vi "Target Detection.vi"(0 "Camera Image":T1) -> (1 "Hot Vision Target":bool, 2 "Cold Vision Target":bool)   [LabVIEW 2013]
uses:
  Support/TargetType.ctl
  <vilib>/vision/Image Controls.llb/IMAQ Image.ctl
panel:
  out "loop time ms":u32
  in  "Instructions:":string="Images:\nUse the tab immediately below to choose the image source. Update the camera settings or the image directory so that you have images or video to test with.\n\nCalibration:\nYou can update Color Component ranges directly, or by clicking and drawing a line on the colored strip in the Image control. The Std Dev multipliers and where the strip is drawn determine the calibration values.\n\nUse Debugging tab to view the result of the color range threshold .\n\nArea Size LImit is used to ignore objects too small or far away to care about.\n\nThe Details tab contains score details for each target and subObject.\n\nCamera Type is used to select lens angles for distance calculation.\n\nVertical strips with no adjacent horizontal strip are identified as \"not hot\" and marked in blue.\nThe numeric scores indicate represent aspect ratio and rectangularity.\n\nWhen both strips are near enough, the pair is identified as \"hot\" and marked in green. Scores\nindicate the left, right, ratio of widths, and vertical positioning.\n\nAny score that falls below cutoff is drawn in red and bounding box is drawn in red."
  in  "Area Size Limit %":dbl=0.06 format="%#_13g"
  in  "Camera Type":enum16{"206", "1011", "1013"}(ring)=enum."1013"
  in  "Score Cutoff":dbl(slide)=54.248366013071895 scale=0.0..100.0
  in  "Color Components":T2={"Hue"={112.0, 144.0}, "Sat"={223.0, 255.0}, "Val"={237.0, 255.0}} {"Val" scale=0.0..255.0; "Sat" scale=0.0..255.0; "Hue" scale=0.0..255.0 scale format="%#_3g"}
  in  "Tabbed Info":enum32{"Debugging", "Details"}(tab)=enum."Details"
  out "Mask":T1(plugin-control)
  out "Target Info":T4(array[cluster])=[{"Scores"={"Total"=264.8428070737725, "Left"=82.00744831503384, "Right"=0.0, "Ratio"=95.56961423095669, "Vertical"=87.265744527782, "index"=0, "State"=enum."Hot"}, "Verticals"={"Horizontal?"=FALSE, "Aspect Score"=83.06845793962944, "Rect Score"=72.28571428571429, {"Left"=200.0, "Top"=96.0, "Right"=207.0, "Bottom"=146.0}, "Equiv H"=5.125465815260874, "Equiv V"=49.36136716524427}, "Horizontals"={"Horizontal?"=TRUE, "Aspect Score"=88.35576607935369, "Rect Score"=66.38655462184875, {"Left"=161.0, "Top"=90.0, "Right"=195.0, "Bottom"=97.0}, "Equiv H"=32.1921978337671, "Equiv V"=4.908021527945207}, "Distance ft"=14.225212029119403, "Center"={"X"=0.271875, "Y"=0.008333333333333333}}]
  out "Image":T1(plugin-control)
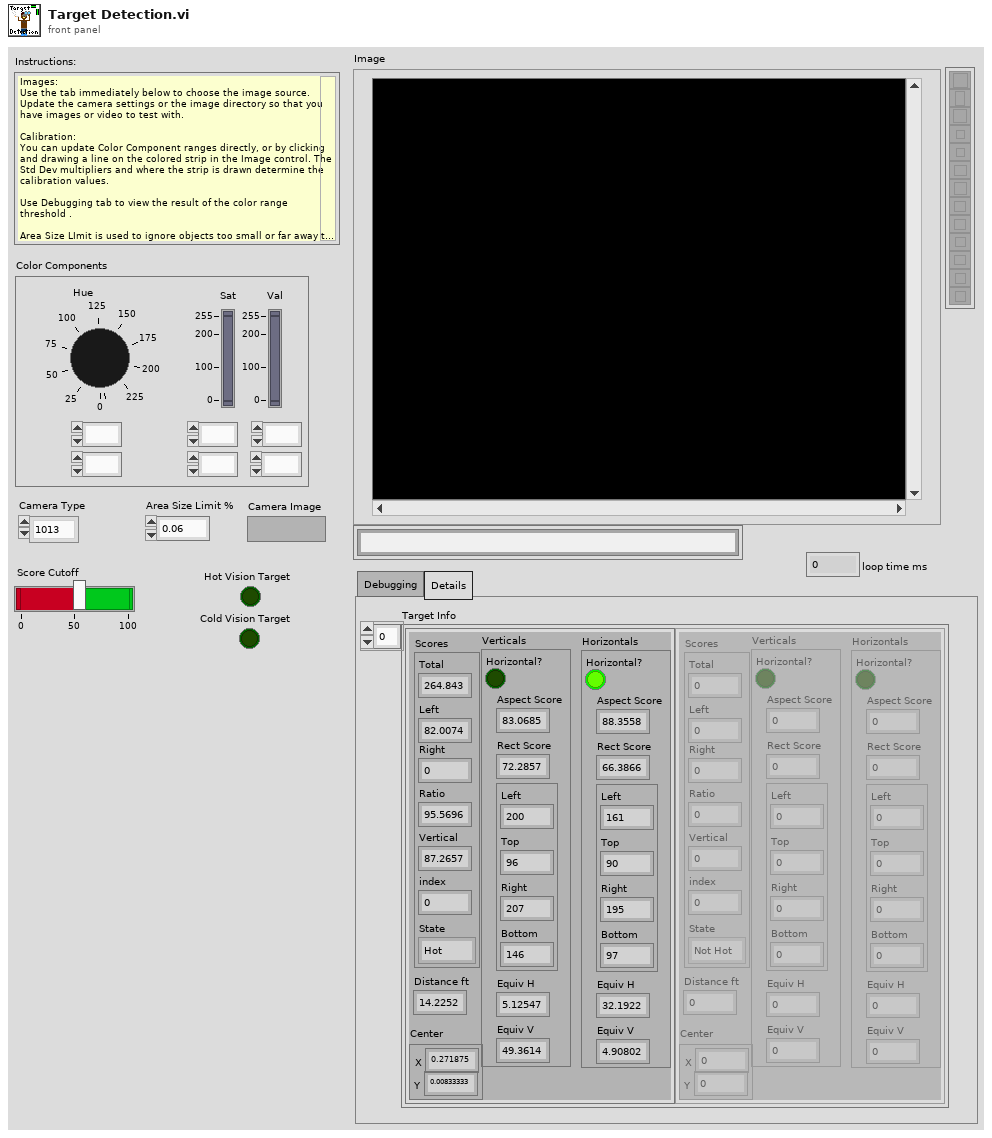
[diagram p1: front panel]
types:
  T1 = typedef "IMAQ Image.ctl" = refnum<image>
  T2 = cluster{"Hue":cluster{dbl, dbl}, "Sat":cluster{dbl, dbl}, "Val":cluster{dbl, dbl}}
  T3 = typedef "TargetType.ctl" = enum16{"Not Hot", "Hot"}
  T4 = cluster{"Scores":cluster{"Total":dbl, "Left":dbl, "Right":dbl, "Ratio":dbl, "Vertical":dbl, "index":i32, "State":T3}, "Verticals":cluster{"Horizontal?":bool, "Aspect Score":dbl, "Rect Score":dbl, cluster{"Left":dbl, "Top":dbl, "Right":dbl, "Bottom":dbl}, "Equiv H":dbl, "Equiv V":dbl}, "Horizontals":cluster{"Horizontal?":bool, "Aspect Score":dbl, "Rect Score":dbl, cluster{"Left":dbl, "Top":dbl, "Right":dbl, "Bottom":dbl}, "Equiv H":dbl, "Equiv V":dbl}, "Distance ft":dbl, "Center":cluster{"X":dbl, "Y":dbl}}[]
  T5 = cluster{"Horizontal":bool, "Aspect Score":dbl, "Rect Score":dbl, cluster{"Left":dbl, "Top":dbl, "Right":dbl, "Bottom":dbl}, "Equiv H":dbl, "Equiv V":dbl}[]
  T6 = cluster{"Scores":cluster{"Total":dbl, "Left":dbl, "Right":dbl, "Ratio":dbl, "Vertical":dbl, "index":i32, "State":T3}, "Verticals":cluster{"Horizontal?":bool, "Aspect Score":dbl, "Rect Score":dbl, cluster{"Left":dbl, "Top":dbl, "Right":dbl, "Bottom":dbl}, "Equiv H":dbl, "Equiv V":dbl}, "Horizontals":cluster{"Horizontal?":bool, "Aspect Score":dbl, "Rect Score":dbl, cluster{"Left":dbl, "Top":dbl, "Right":dbl, "Bottom":dbl}, "Equiv H":dbl, "Equiv V":dbl}, "Validated":bool}[]
  T7 = cluster{"Scores":cluster{"Total":dbl, "Left":dbl, "Right":dbl, "Ratio":dbl, "Vertical":dbl, "index":i32, "State":T3}, "Verticals":cluster{"Horizontal?":bool, "Aspect Score":dbl, "Rect Score":dbl, cluster{"Left":dbl, "Top":dbl, "Right":dbl, "Bottom":dbl}, "Equiv H":dbl, "Equiv V":dbl}, "Horizontals":cluster{"Horizontal?":bool, "Aspect Score":dbl, "Rect Score":dbl, cluster{"Left":dbl, "Top":dbl, "Right":dbl, "Bottom":dbl}, "Equiv H":dbl, "Equiv V":dbl}, "Distance (ft)":dbl, "Target Center (-1 to 1)":cluster{"X":dbl, "Y":dbl}}[]
  T8 = cluster{"Scores":cluster{"Total":dbl, "Left":dbl, "Right":dbl, "Ratio":dbl, "Vertical":dbl, "index":i32, "State":T3}, "Verticals":cluster{"Horizontal?":bool, "Aspect Score":dbl, "Rect Score":dbl, cluster{"Left":dbl, "Top":dbl, "Right":dbl, "Bottom":dbl}, "Equiv H":dbl, "Equiv V":dbl}, "Horizontals":cluster{"Horizontal?":bool, "Aspect Score":dbl, "Rect Score":dbl, cluster{"Left":dbl, "Top":dbl, "Right":dbl, "Bottom":dbl}, "Equiv H":dbl, "Equiv V":dbl}, "Distance (ft)":dbl, "Target Center (-1 to 1)":cluster{"X":dbl, "Y":dbl}}
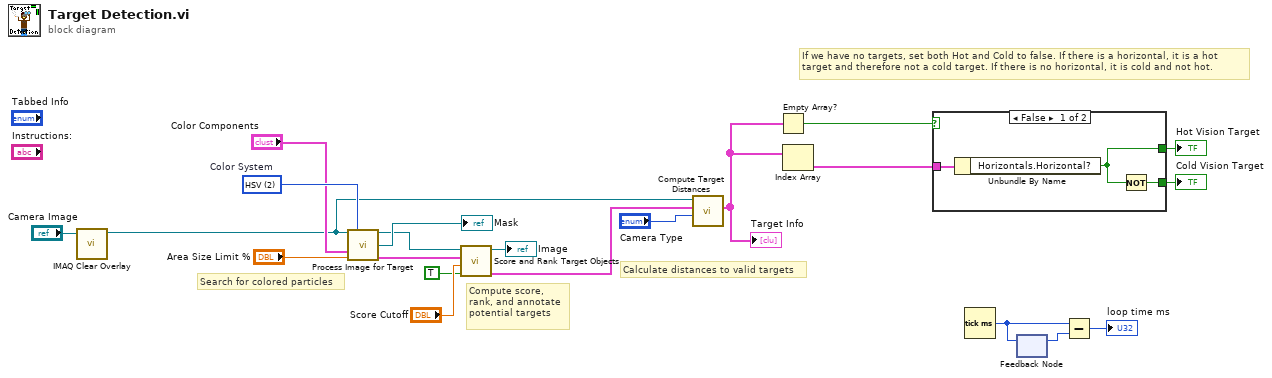
[diagram p0: block diagram]
diagram:
  w13 = u16 2 items=["RGB", "HSL", "HSV", "HSI"]  # Color System
  # "If we have no targets, set both Hot and Cold to false. If there is a horizontal, it is a hot\ntarget and therefore not a cold target. If there is no horizontal, it is cold and not hot."
  # "Calculate distances to valid targets"
  # "Search for colored particles"
  # "Compute score,\nrank, and annotate\npotential targets"
  n1 = call "IMAQ Clear Overlay"("Image"="Camera Image") -> ("Image Out"=w11:T1)  [unwired: 9 in, 1 out]
  n2 = call "Process Image for Target.vi"("Src Image"=w11, "Color Mode"=w13, "Color Components"="Color Components", "Area Cutoff %"="Area Size Limit %") -> ("Src Image Out"=w19:T1, "Threshold"=→"Mask":T1, "Particles"=w16:T5)  [unwired: 9 in]
  n3 = call "Score and Rank Target Objects.vi"("Annotate"=TRUE, "Score Limit"="Score Cutoff", "Particles"=w16, "Image in"=w19) -> ("Target Info"=w15:T6, "Annotated Image"=→"Image":T1)  [unwired: 6 in]
  n4 = call "Compute Target Distances.vi"("Camera Type"="Camera Type", "Target Info"=w15, "Image in"=w11) -> ("Target Info"=w6:T7)  [unwired: 6 in, 2 out]
  "Target Info" <- w6
  n5 = Empty Array?(array=w6) -> (empty?=w7:bool)
  n6 = Index Array(array=w6) -> (element=w8:T8)  [unwired: 1 in]
  n7 = case shown="False" w7 {
    tunnel: w8 -> [w24 _]
    tunnel: [w23 _] -> w2
    tunnel: [w22 _] -> w1
    frame False {
      n8 = Unbundle By Name(w24) -> ("Horizontals.Horizontal?"=w23:bool)
      n9 = Not(x=w23) -> (.not. x?=w22:bool)
    }
    frame True {
    }
  }
  "Hot Vision Target" <- w2
  "Cold Vision Target" <- w1
  n10 = Tick Count (ms)() -> (millisecond timer value=w5:u32)
  n11 = feedback #1() -> (w4:u32)  [unwired: 1 in]
  n12 = feedback-in #1(w5) -> ()
  n13 = Subtract(x=w5, y=w4) -> (x-y=→"loop time ms":u32)
